vi "DashboardLEDStatesBack.vi"(0 "Default":string, 1 "State":string, 2 "Traction":string, 3 "Gear Ready":string, 4 "Gear Loaded":string, 5 "Break On":string) -> (6 "RED":bool, 7 "GREEN":bool, 8 "BLUE":bool)   [LabVIEW 2016]
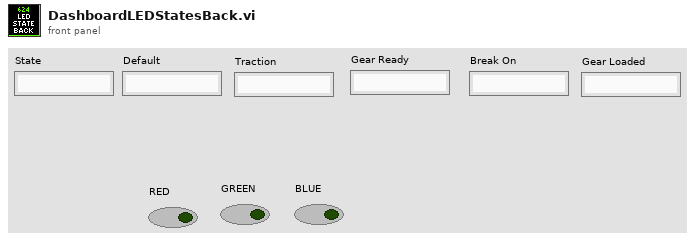
[diagram p1: front panel]
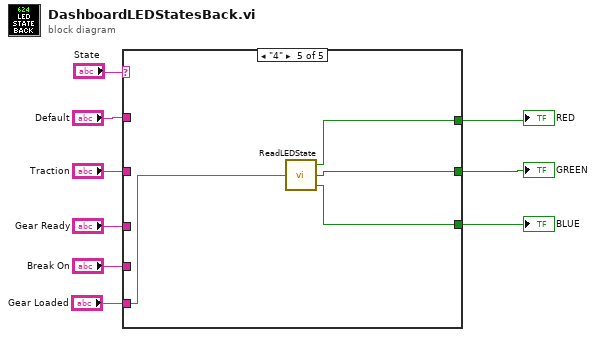
[diagram p0: block diagram]
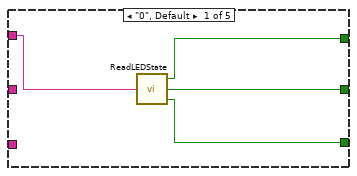
[diagram p2: hidden frame]
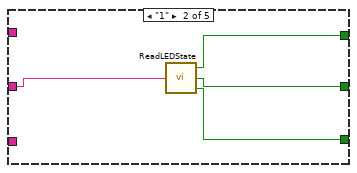
[diagram p3: hidden frame]
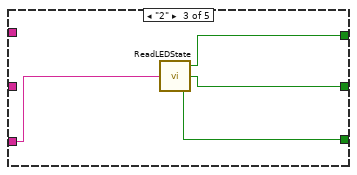
[diagram p4: hidden frame]
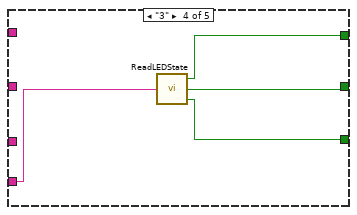
[diagram p5: hidden frame]
diagram:
  n1 = case shown="\"4\"" "State" {
    tunnel: "Default" -> [w13 _ _ _ _]
    tunnel: "Traction" -> [_ w17 _ _ _]
    tunnel: "Gear Ready" -> [_ _ w18 _ _]
    tunnel: [w12 w16 w21 w25 w28] -> w6
    tunnel: [w11 w15 w20 w24 w27] -> w7
    tunnel: [w10 w14 w19 w23 w26] -> w8
    tunnel: "Break On" -> [_ _ _ w22 _]
    tunnel: "Gear Loaded" -> [_ _ _ _ w29]
    frame "0", Default {
      n2 = call "ReadLEDState.vi"("State"=w13) -> ("BLUE"=w10:bool, "GREEN"=w11:bool, "RED"=w12:bool)  [unwired: 2 in]
    }
    frame "1" {
      n3 = call "ReadLEDState.vi"("State"=w17) -> ("BLUE"=w14:bool, "GREEN"=w15:bool, "RED"=w16:bool)  [unwired: 2 in]
    }
    frame "2" {
      n4 = call "ReadLEDState.vi"("State"=w18) -> ("BLUE"=w19:bool, "GREEN"=w20:bool, "RED"=w21:bool)  [unwired: 2 in]
    }
    frame "3" {
      n5 = call "ReadLEDState.vi"("State"=w22) -> ("BLUE"=w23:bool, "GREEN"=w24:bool, "RED"=w25:bool)  [unwired: 2 in]
    }
    frame "4" {
      n6 = call "ReadLEDState.vi"("State"=w29) -> ("BLUE"=w26:bool, "GREEN"=w27:bool, "RED"=w28:bool)  [unwired: 2 in]
    }
  }
  "RED" <- w6
  "GREEN" <- w7
  "BLUE" <- w8
